vi "Aliased Tone Tracker.vi"(7 "sampling frequency":dbl format="%0.2p", 11 "real tone frequency":dbl format="%0.2p") -> (3 "aliased tone frequency":dbl format="%0.2p")   [LabVIEW 2020, in "NI_MAPro.lvlib"]
uses:
  NI_MAPro.lvlib
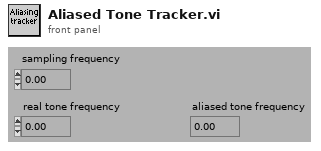
[diagram p1: front panel]
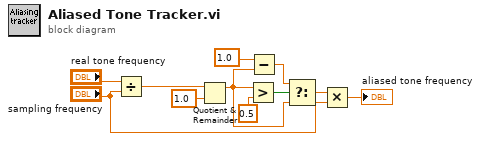
[diagram p0: block diagram]
diagram:
  n1 = Divide(x="real tone frequency", y="sampling frequency") -> (x/y=w10:dbl)
  n2 = Quotient & Remainder(x=w10, y=1.0) -> (x-y*floor(x/y)=w4:dbl)  [unwired: 1 out]
  n3 = Greater?(x=w4, y=0.5) -> (0:w7:bool)
  n4 = Subtract(x=1.0, y=w4) -> (x-y=w5:dbl)
  n5 = Select(t=w5, s=w7, f=w4) -> (s? t:f=w3:dbl)
  n6 = Multiply(x=w3, y="sampling frequency") -> (x*y=→"aliased tone frequency":dbl)
